vi "Test CAN Logger with TDMS.vi"() -> ()   [LabVIEW 2014]
uses:
  <vilib>/RioEmbeddedCAN/RioEmbeddedCAN.llb/CANFrameControl.ctl
  Formula Hybrid 2012 r1/CAN/8byte to 4 2byte.vi
  Formula Hybrid 2012 r1/CAN/TDMS Timestamp and Data.vi
  Formula Hybrid 2012 r1/CAN/Decode VSM.vi
  Formula Hybrid 2012 r1/CAN/Decode Inverter State.vi
  Formula Hybrid 2012 r1/CAN/Decode Inverter Enable States.vi
  Formula Hybrid 2012 r1/CAN/Decode Inverter Command Modes.vi
  Formula Hybrid 2012 r1/CAN/BMS/Decode Car State.vi
  Formula Hybrid 2012 r1/CAN/BMS/Scale Cell Voltage.vi
  Formula Hybrid 2012 r1/CAN/BMS/Scale Cell Temp.vi
  Formula Hybrid 2012 r1/Global Data.vi
  Formula Hybrid 2012 r1/CAN/BMS/Decode Charging State.vi
panel:
  out "Array":cluster{"CAN frame":T1, "timestamp":timestamp}[](array[cluster]) {"CAN frame"."type" items=["CAN Data", "CAN Remote"]; "CAN frame"."identifier" format="%.0x"}
  in  "Stop Frame Collection":bool
  out "error out":errorcluster
  out "index":i32
  in  "baud rate (125000 bps)":u32=1000000
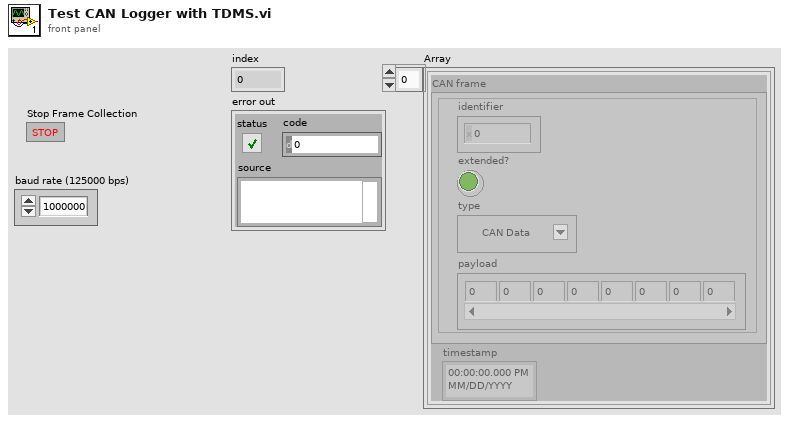
[diagram p1: front panel]
types:
  T1 = typedef "CANFrameControl.ctl" = cluster{"identifier":u32, "extended?":bool, "type":u8, "payload":u8[]}
  T2 = enum16{"open", "open or create", "create or replace", "create", "open (read-only)"}
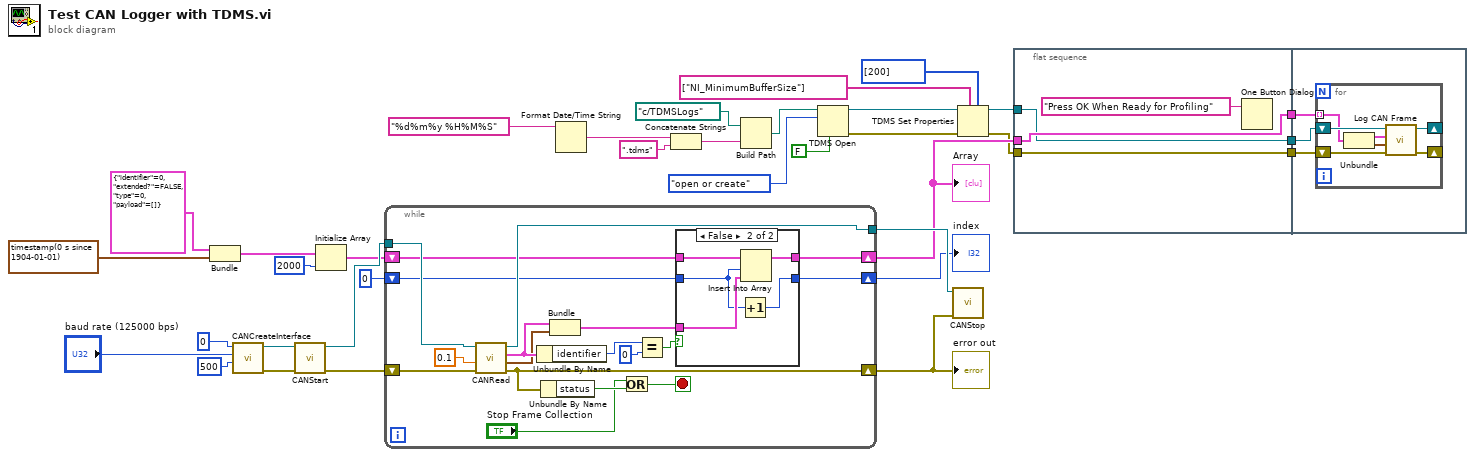
[diagram p0: block diagram]
diagram:
  n1 = Bundle("CAN frame"=T1 {"identifier"=0, "extended?"=FALSE, "type"=0, "payload"=[]}, "timestamp"=timestamp(0 s since 1904-01-01)) -> (w7:cluster{"CAN frame":T1, "timestamp":timestamp})  [unwired: 1 in]
  n2 = call <vilib>:"CANCreateInterface.vi"("receive queue size (5)"=u32 500, "baud rate (125000 bps)"="baud rate (125000 bps)", "interface index"=u32 0) -> ("error out"=w34:errorcluster, "interface object out"=w33:refnum<k20>)  [unwired: 7 in]
  n3 = call <vilib>:"CANStart.vi"("error in (no error)"=w34, "interface object in"=w33) -> ("error out"=w24:errorcluster, "interface object out"=w32:refnum<k20>)  [unwired: 8 in]
  n4 = Initialize Array(w7, 2000 ("dimension size")) -> (w27:cluster{"CAN frame":T1, "timestamp":timestamp}[])
  n5 = while {
    tunnel: w32 -> [w52]
    tunnel: [w51] -> w31
    shift-right: [w44] -> w6
    shift-left: w27 -> [w50]
    shift-right: [w45] -> w22
    shift-left: 0 ("index") -> [w49]
    shift-right: [w41] -> w30
    shift-left: w24 -> [w42]
    stop <- w40 stop-if-true
    n6 = call <vilib>:"CANRead.vi"("error in (no error)"=w42, "timeout (0 s)"=0.1, "interface object in"=w52) -> ("error out"=w41:errorcluster, "timestamp"=w36:timestamp, "CAN frame"=w37:T1, "interface object out"=w51:refnum<k20>)  [unwired: 5 in]
    n7 = Unbundle By Name(w37) -> ("identifier"=w48:u32)
    n8 = Unbundle By Name(w41) -> ("status"=w39:bool)
    n9 = Bundle("CAN frame"=w37, "timestamp"=w36) -> (w35:cluster{"CAN frame":T1, "timestamp":timestamp})  [unwired: 1 in]
    n10 = Or(x="Stop Frame Collection", y=w39) -> (x .or. y?=w40:bool)
    n11 = Equal?(x=w48, y=u32 0) -> (x = y?=w46:bool)
    n12 = case shown="False" w46 {
      tunnel: w50 -> [w54 w59]
      tunnel: [w54 w58] -> w44
      tunnel: w49 -> [w53 w56]
      tunnel: w35 -> [_ w57]
      tunnel: [w53 w55] -> w45
      frame True {
      }
      frame False {
        n13 = Increment(x=w56) -> (x+1=w55:i32)
        n14 = Insert Into Array(array=w59, index=w56, new element=w57) -> (w58:cluster{"CAN frame":T1, "timestamp":timestamp}[])
      }
    }
  }
  "index" <- w22
  "error out" <- w30
  "Array" <- w6
  n15 = Format Date/Time String(time format string (%c)="%d%m%y %H%M%S") -> (date/time string=w18:string)  [unwired: 2 in]
  n16 = Concatenate Strings(w18, ".tdms" ("string")) -> (w20:string)
  n17 = Build Path(base path=path "c:/TDMSLogs", name or relative path=w20) -> (appended path=w19:path)
  n18 = TDMS Open(6:FALSE ("disable buffering? (T)"), 10:T2."open or create" ("operation (0:open)"), 11:w19) -> (0:w13:errorcluster, 3:w12:refnum<k34>)  [unwired: 4 in]
  n19 = call <vilib>:"CANStop.vi"("error in (no error)"=w30, "interface object in"=w31) -> ()  [unwired: 8 in, 2 out]
  n20 = TDMS Set Properties(5:i32[] [200] ("property values"), 7:string[] ["NI_MinimumBufferSize"] ("property names"), 8:w13, 11:w12) -> (0:w4:errorcluster, 3:w5:refnum<k34>)  [unwired: 2 in, 2 out]
  n21 = flat-sequence {
    tunnel: w4 -> [w61]
    tunnel: w5 -> [w62]
    tunnel: w6 -> [w63]
    tunnel: [w63] -> w3
    tunnel: [w62] -> w2
    tunnel: [w61] -> w1
    tunnel: w3 -> [w66]
    tunnel: w2 -> [w65]
    tunnel: w1 -> [w64]
    frame #0 {
      n22 = One Button Dialog(message="Press OK When Ready for Profiling") -> ()  [unwired: 1 in, 1 out]
    }
    frame #1 {
      n23 = for {
        tunnel: w66 -> [w71] mode=indexing
        shift-right: [w68] -> _
        shift-left: w65 -> [w73]
        shift-right: [w67] -> _
        shift-left: w64 -> [w72]
        n24 = Unbundle(w71) -> ("CAN frame"=w69:T1, "timestamp"=w70:timestamp)
        n25 = call "Log CAN Frame.vi"("error in (no error)"=w72, "timestamp"=w70, "CAN frame"=w69, "tdms file"=w73) -> ("error out"=w67:errorcluster, "tdms file out"=w68:refnum<k34>)  [unwired: 6 in]
      }
    }
  }
